vi "Speaker Output Test.vi"(9 "Simulation Data":T1={"PowerOn"=TRUE, "Battery"=TRUE, "Antenna"=TRUE, "Microphone"=TRUE, "Speakers"=TRUE, "Buttons"=TRUE, "LCD"=enum."Passing Image"}, 10 "High Frequency":dbl=40000.0 format="%0.2f", 11 "Low Frequency":dbl=1000.0 format="%0.2f") -> (0 "error out":errorcluster, 2 "Frequency Response":dbl[][](array[numeric]), 3 "Minimum Amplitude":dbl)   [LabVIEW 2011]
doc: "Measures the Test fixture microphone input while a frequency sweep test sound is played by the speaker on the UUT. The amplitude of the response is measured to ensure that the UUT speaker is playing all pitches in the desired frequency range. The Test returns the minimum measured amplitude of all tested frequencies."
uses:
  Support/Simulation Data.ctl
  <vilib>/Analysis/1siggen.llb/Ramp Pattern by Samples.vi
  <vilib>/Analysis/NI_AALBase.lvlib
panel:
  out "Amplitude Plot":cluster{dbl[], dbl[]}(graph)
  # "Settings"
  # "Results"
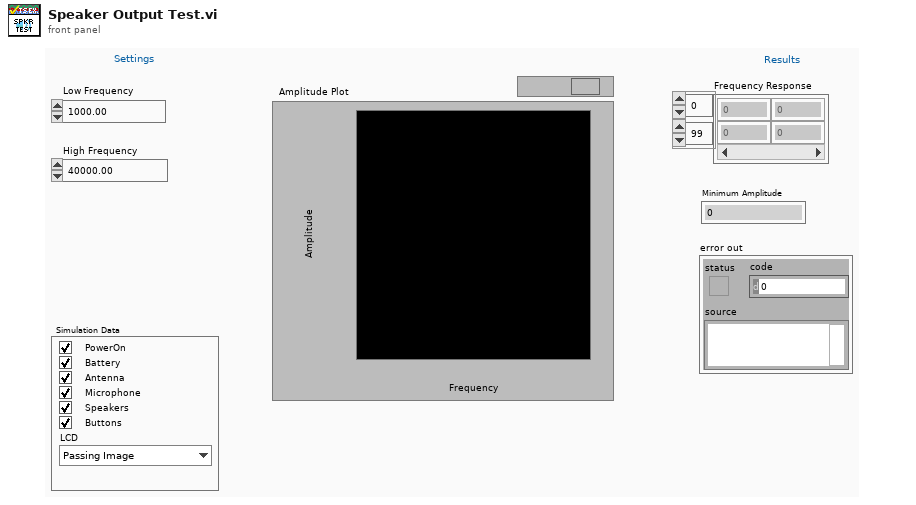
[diagram p1: front panel]
types:
  T1 = typedef "Simulation Data.ctl" = cluster{"PowerOn":bool, "Battery":bool, "Antenna":bool, "Microphone":bool, "Speakers":bool, "Buttons":bool, "LCD":enum16{"Passing Image", "Dead Pixels", "Incorrect Brightness"}}
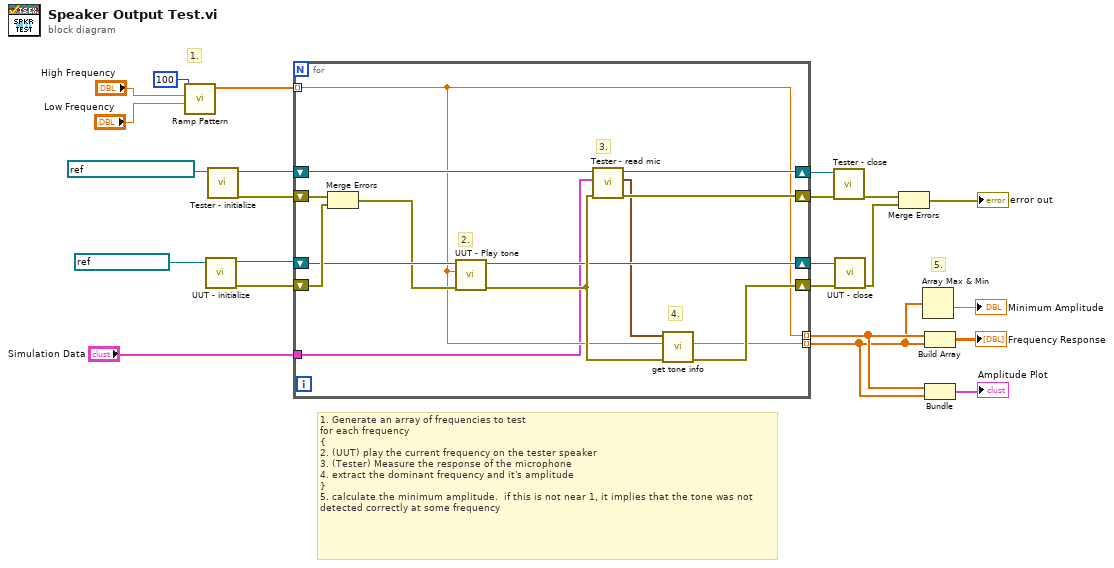
[diagram p0: block diagram]
diagram:
  # "5."
  # "1."
  # "1. Generate an array of frequencies to test\nfor each frequency\n{\n2. (UUT) play the current frequency on the tester speaker\n3. (Tester) Measure the response of the microphone\n4. extract the dominant frequency and it's amplitude\n}\n5. calculate the minimum amplitude.  if this is not near 1, it implies that the tone was not detected correctly at some frequency"
  n1 = call-poly <vilib>:"Ramp Pattern.vi"("start"="Low Frequency", "end"="High Frequency", "samples"=100) -> ("Ramp Pattern"=w20:dbl[])  [unwired: 7 in, 1 out]
  n2 = call "UUT - initialize.vi"("VISA resource name"=refnum<visa-resource-name> "UUTController") -> ("error out"=w16:errorcluster, "VISA resource name out"=w14:refnum<visa-resource-name>)  [unwired: 9 in]
  n3 = call "Tester - initialize.vi"("VISA resource name"=refnum<visa-resource-name> "TesterAudioMeasure") -> ("error out"=w15:errorcluster, "VISA resource name out"=w13:refnum<visa-resource-name>)  [unwired: 9 in]
  n4 = for {
    shift-right: [w37] -> w11
    shift-left: w16 -> [w35]
    tunnel: [w25] -> w4 mode=indexing
    tunnel: [w26] -> w3 mode=indexing
    tunnel: w20 -> [w25] mode=indexing
    shift-right: [w31] -> w10
    shift-left: w15 -> [w36]
    shift-right: [w30] -> w9
    shift-left: w13 -> [w29]
    shift-right: [w28] -> w8
    shift-left: w14 -> [w34]
    tunnel: "Simulation Data" -> [w24]
    # "4."
    # "3."
    # "2."
    n5 = Merge Errors(w36, w35) -> (w33:errorcluster)
    n6 = call "UUT - Play tone.vi"("error in (no error)"=w33, "Frequency"=w25, "VISA resource name"=w34) -> ("error out"=w32:errorcluster, "VISA resource name out"=w28:refnum<visa-resource-name>)  [unwired: 7 in]
    n7 = call "Tester - read mic.vi"("error in (no error)"=w32, "Simulation Data"=w24, "VISA resource name"=w29) -> ("error out"=w31:errorcluster, "Response Signal Out"=w27:waveform(dbl), "VISA resource name out"=w30:refnum<visa-resource-name>)  [unwired: 6 in]
    n8 = call "get tone info.vi"("error in (no error)"=w32, "Expected Frequency"=w25, "time signal in"=w27) -> ("error out"=w37:errorcluster, "Amplitude"=w26:dbl)  [unwired: 6 in, 1 out]
  }
  n9 = call "Tester - close.vi"("error in (no error)"=w10, "VISA resource name"=w9) -> ("error out"=w6:errorcluster)  [unwired: 9 in]
  n10 = call "UUT - close.vi"("error in (no error)"=w11, "VISA resource name"=w8) -> ("error out"=w7:errorcluster)  [unwired: 9 in]
  n11 = Merge Errors(w6, w7) -> (→"error out":errorcluster)
  n12 = Array Max & Min(array=w3) -> (min value=→"Minimum Amplitude":dbl)  [unwired: 3 out]
  n13 = Build Array(w4, w3) -> (→"Frequency Response":dbl[][])
  n14 = Bundle(w4, w3) -> (→"Amplitude Plot":cluster{dbl[], dbl[]})  [unwired: 1 in]
